vi "Initialize.vi"(8 "error in (no error)":errorcluster, 9 "Serial Configuration":T1={"Baud Rate"=115200, "Parity"=0, "Data Bits"=8, "Stop Bits"=10, "Flow Control"=0} {"Flow Control" items=["None", "XON/XOFF", "RTS/CTS", "XON/XOFF & RTS/CTS", "DTR/DSR", "XON/XOFF & DTR/DSR"]; "Stop Bits" items=["1.0"=10, "1.5"=15, "2.0"=20]; "Data Bits" items=["7"=7, "8"=8]; "Parity" items=["None", "Odd", "Even", "Mark", "Space"]; "Baud Rate" items=["300"=300, "600"=600, "1200"=1200, "2400"=2400, "4800"=4800, "9600"=9600, "19200"=19200, "115200"=115200]}, 10 "Reset (True)":bool=TRUE, 11 "VISA resource name":refnum<visa-resource-name>) -> (0 "error out":errorcluster, 3 "VISA resource name out":refnum<visa-resource-name>)   [LabVIEW 2013, in "Watts Up PRO Net Series.lvlib"]
doc: "Establishes communication with the instrument and optionally performs an instrument identification query and/or an instrument reset. It also places the instrument in a default state needed for other instrument driver operations. Therefore, call this VI before calling other instrument driver VIs for this instrument. Generally, you need to call the <b>Initialize</b> VI only once at the beginning of an application."
uses:
  <instrlib>/Watts Up PRO Net Series/Watts Up PRO Net Series.lvlib
panel:
  # "(c) 2014 NATIONAL INSTRUMENTS.  ALL RIGHTS RESERVED."
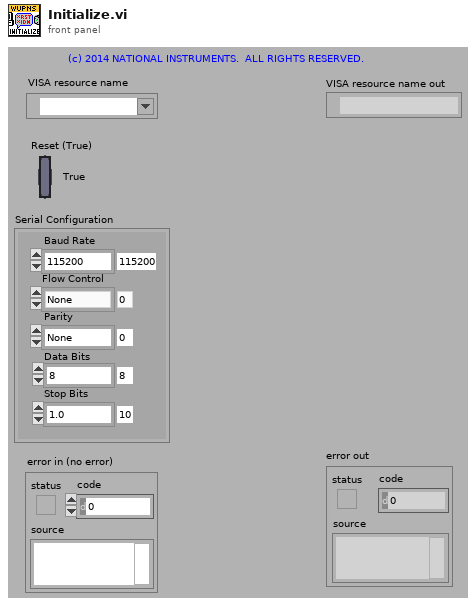
[diagram p1: front panel]
types:
  T1 = cluster{"Baud Rate":u32, "Parity":u16, "Data Bits":u16, "Stop Bits":u16, "Flow Control":u16}
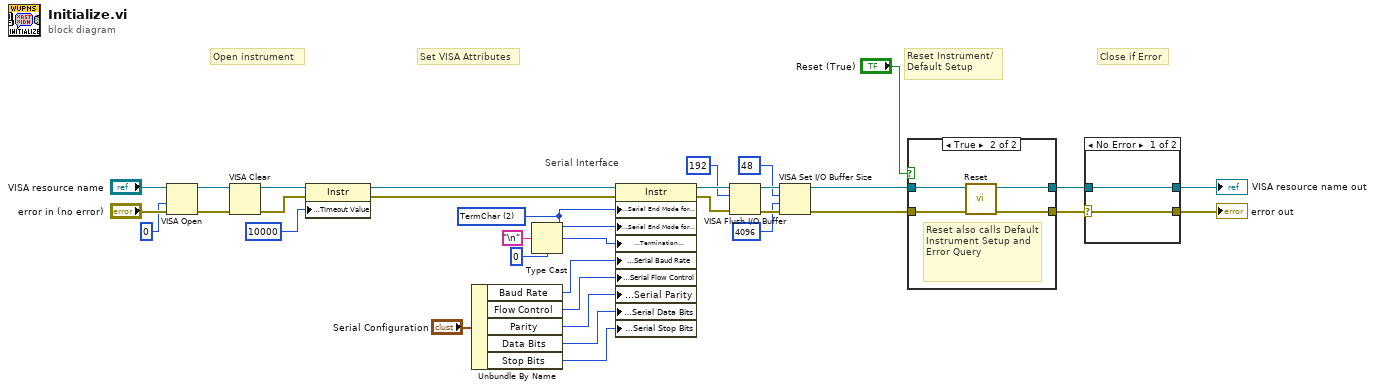
[diagram p0: block diagram]
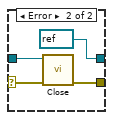
[diagram p2: hidden frame]
diagram:
  w9 = u16 2 items=["None", "LastBit", "TermChar"] ("Serial Settings:Serial End Mode for Reads")
  # "Serial Interface"
  # "Set VISA Attributes"
  # "Close if Error"
  # "Reset Instrument/\nDefault Setup"
  # "Open instrument"
  n1 = VISA Open(access mode=u32 0, error in (no error)="error in (no error)", VISA resource name="VISA resource name") -> (VISA resource name=w27:refnum<visa-resource-name>, error out=w26:errorcluster)  [unwired: 2 in]
  n2 = VISA Clear(VISA resource name=w27, error in (no error)=w26) -> (VISA resource name out=w25:refnum<visa-resource-name>, error out=w24:errorcluster)
  n3 = property class="Instr"(reference=w25, error in=w24, "General Settings:Timeout Value"=u32 10000) -> (reference out=w30:refnum<visa-resource-name>, error out=w29:errorcluster)
  n4 = Unbundle By Name("Serial Configuration") -> ("Baud Rate"=w7:u32, "Flow Control"=w3:u16, "Parity"=w5:u16, "Data Bits"=w6:u16, "Stop Bits"=w2:u16)
  n5 = Type Cast(type=u8 0, x="\n" ("Line Feed Constant")) -> (*(type *) &x=w8:u8)
  n6 = property class="Instr"(reference=w30, error in=w29, "Serial Settings:Serial End Mode for Reads"=w9, "Serial Settings:Serial End Mode for Writes"=w9, "Message Based Settings:Termination Character"=w8, "Serial Settings:Serial Baud Rate"=w7, "Serial Settings:Serial Flow Control"=w3, "Serial Settings:Serial Parity"=w5, "Serial Settings:Serial Data Bits"=w6, "Serial Settings:Serial Stop Bits"=w2) -> (reference out=w15:refnum<visa-resource-name>, error out=w17:errorcluster)
  n7 = VISA Flush I/O Buffer(VISA resource name=w15, mask (16)=u16 192, error in (no error)=w17) -> (VISA resource name out=w18:refnum<visa-resource-name>, error out=w16:errorcluster)
  n8 = VISA Set I/O Buffer Size(VISA resource name=w18, mask (16)=u16 48, size (4096)=u32 4096 ("size (0)"), error in (no error)=w16) -> (VISA resource name out=w20:refnum<visa-resource-name>, error out=w19:errorcluster)
  n9 = case shown="True" "Reset (True)" {
    tunnel: [w35 w40] -> w21
    tunnel: [w36 w39] -> w22
    tunnel: w20 -> [w36 w38]
    tunnel: w19 -> [w35 w37]
    frame False {
    }
    frame True {
      # "Reset also calls Default Instrument Setup and Error Query"
      n10 = call <instrlib>:"Reset.vi"("error in (no error)"=w37, "VISA resource name"=w38) -> ("error out"=w40:errorcluster, "VISA resource name out"=w39:refnum<visa-resource-name>)  [unwired: 8 in]
    }
  }
  n11 = case shown="No Error" w21 {
    selector: w21 -> [w41 w44]
    tunnel: w22 -> [w42 w45]
    tunnel: [w42 refnum<visa-resource-name> refnum ("VISA resource name out")] -> w23
    tunnel: [w41 w46] -> w1
    frame No Error {
    }
    frame Error {
      n12 = call <instrlib>:"Close.vi"("error in (no error)"=w44, "VISA resource name"=w45) -> ("error out"=w46:errorcluster)  [unwired: 9 in]
    }
  }
  "VISA resource name out" <- w23
  "error out" <- w1
